vi "Instrument fgv.vi"(7 "Enum":T1(ring), 8 "error in (no error) 2":errorcluster, 10 "WriteCC1":string[](array[string])=[""], 11 "INPUT":T2) -> (0 "error":errorcluster, 2 "WriteCC1 2":string[](array[string]), 3 "output":T2)   [LabVIEW 2025]
uses:
  40ab9981-9a43-4b6a-897e-d3960d716397.vi
  <vilib>/Utility/error.llb/Trim Whitespace One-Sided.vi
  <vilib>/Instr/_visa.llb/VISA Configure Serial Port (Instr).vi
panel:
  out "trimmed string":string
  out "error out 3":errorcluster
  out "error out":errorcluster
  out "Serial Settings:Number of Bytes at Serial Port":u32
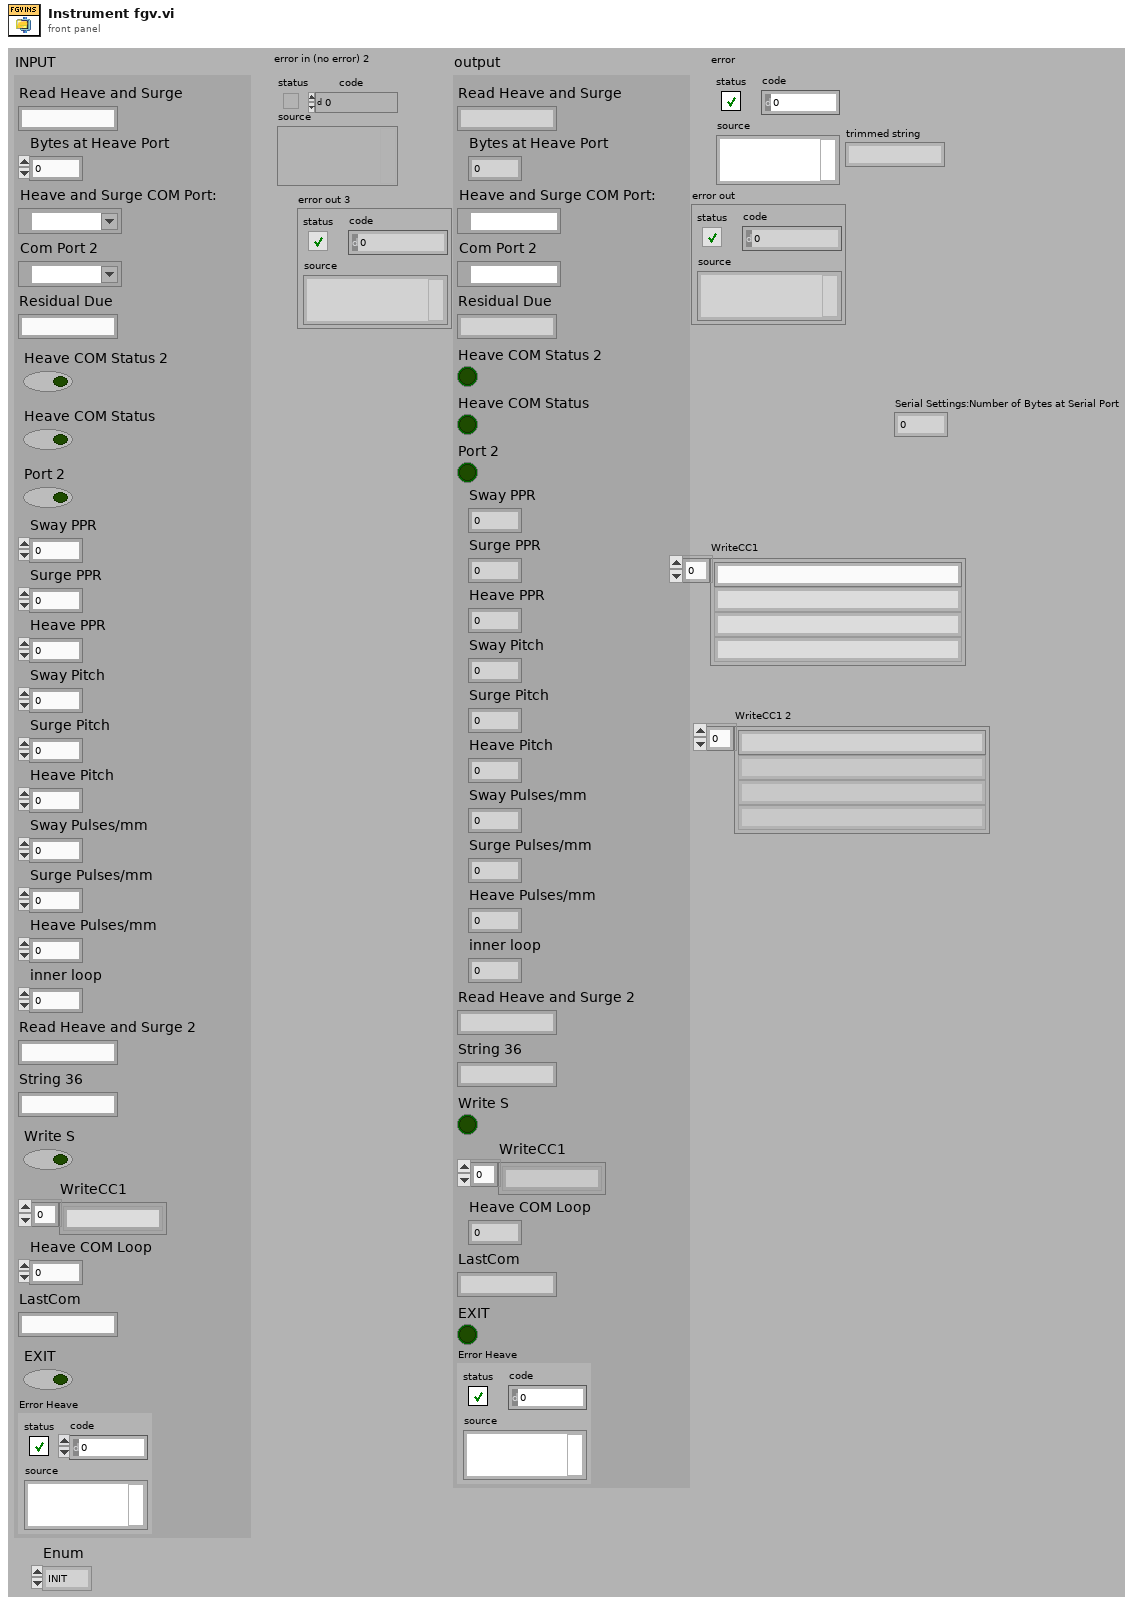
[diagram p1: front panel]
types:
  T1 = enum16{"INIT", "READ", "MANUAL WRITE", "WRITE", "CLOSE", "ERROR INIT"}
  T2 = cluster{"Read Heave and Surge":string, "Bytes at Heave Port":dbl, "Heave and Surge COM Port:":refnum<visa-resource-name>, "Com Port 2":refnum<visa-resource-name>, "Residual Due":string, "Heave COM Status 2":bool, "Heave COM Status":bool, "Port 2":bool, "Sway PPR":dbl, "Surge PPR":dbl, "Heave PPR":dbl, "Sway Pitch":dbl, "Surge Pitch":dbl, "Heave Pitch":dbl, "Sway Pulses/mm":dbl, "Surge Pulses/mm":dbl, "Heave Pulses/mm":dbl, "inner loop":dbl, "Read Heave and Surge 2":string, "String 36":string, "Write S":bool, "WriteCC1":string[], "Heave COM Loop":i32, "LastCom":string, "EXIT":bool, "Error Heave":errorcluster}
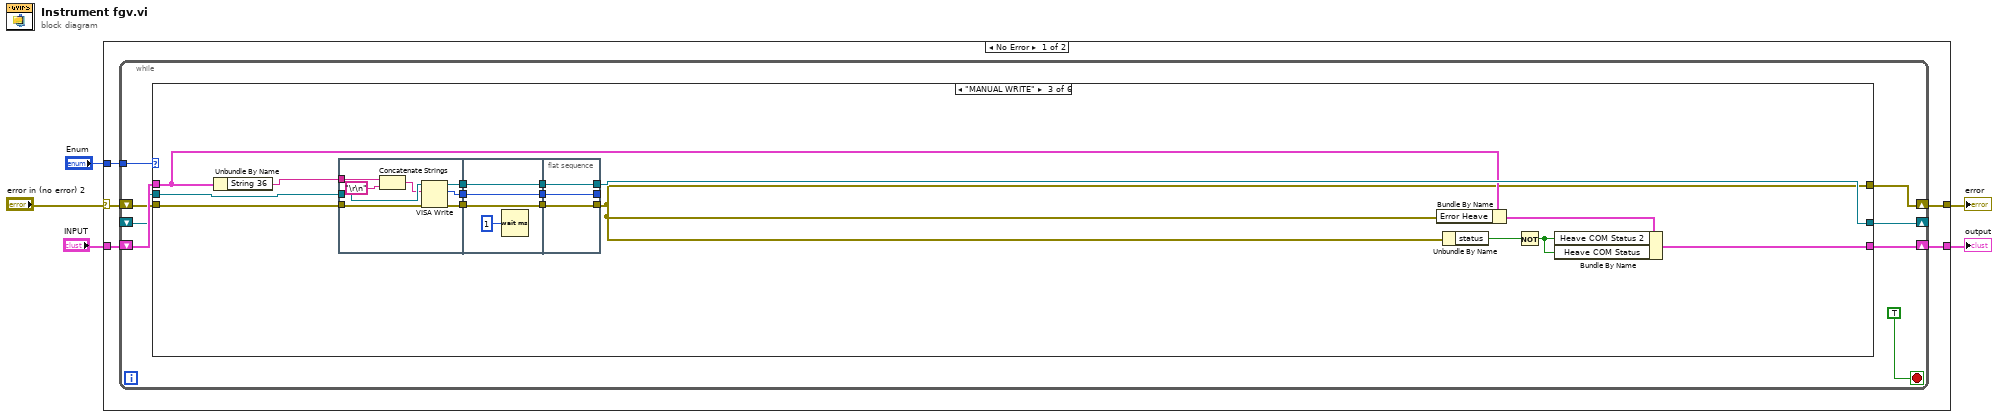
[diagram p0: block diagram]
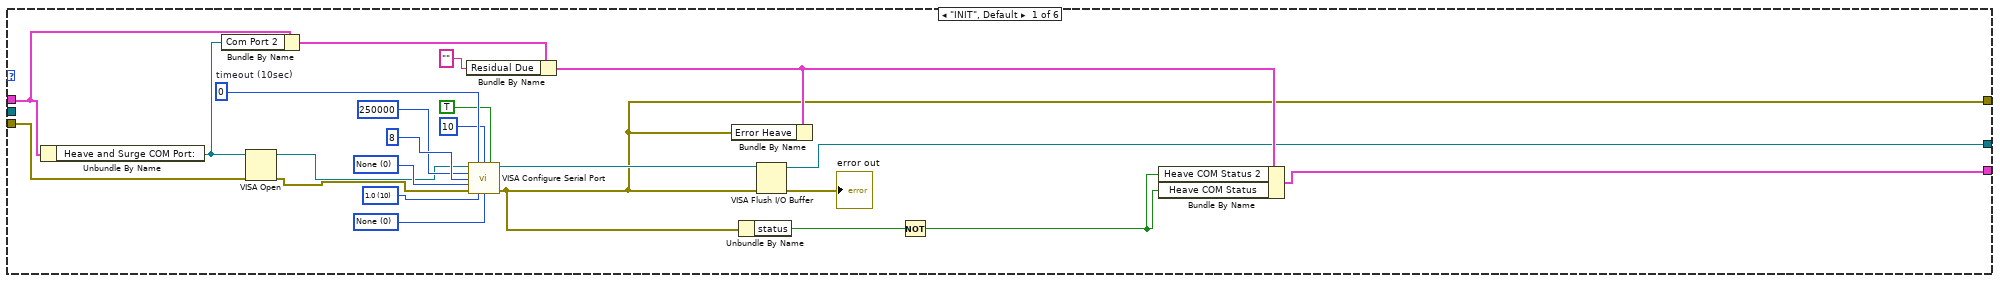
[diagram p2: hidden frame]
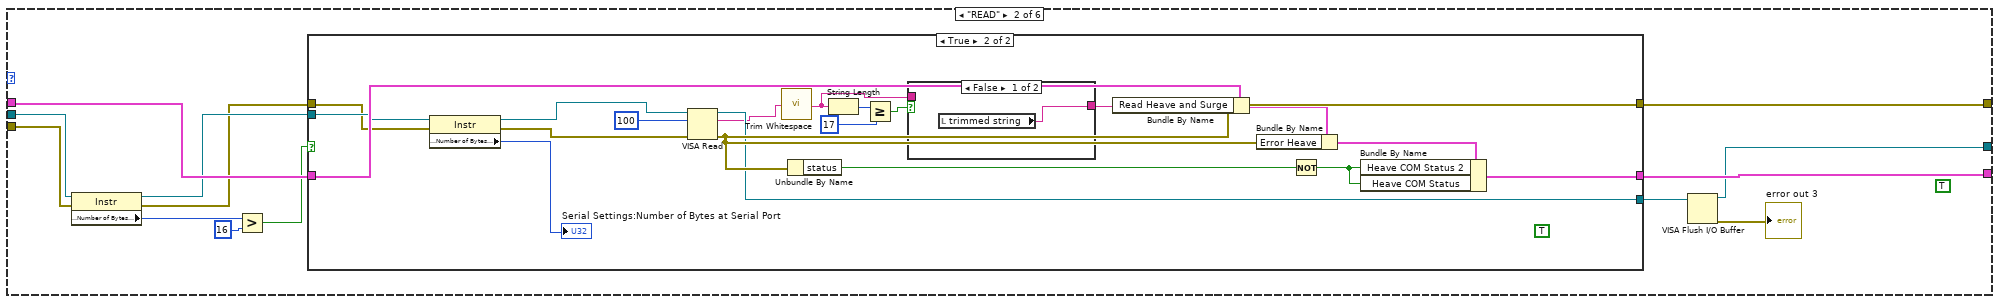
[diagram p3: hidden frame]
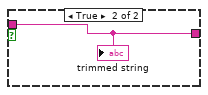
[diagram p5: hidden frame]
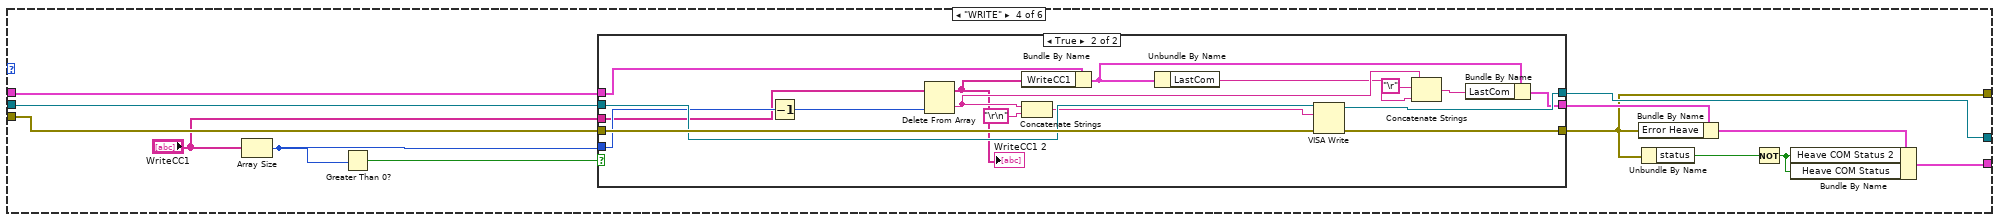
[diagram p6: hidden frame]
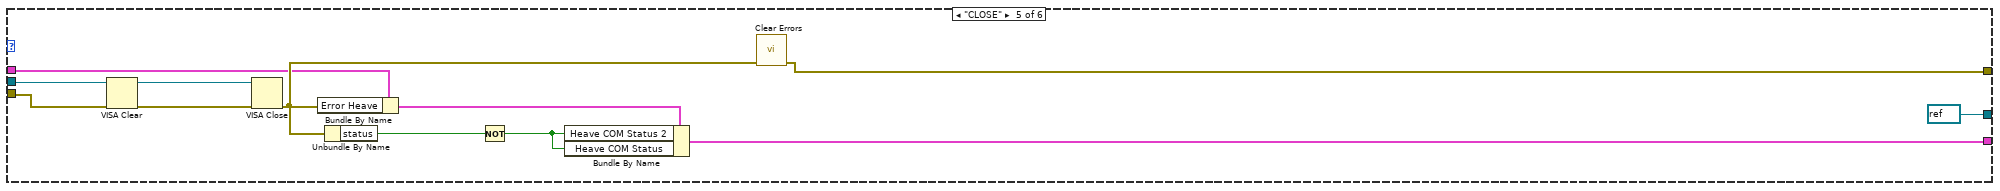
[diagram p8: hidden frame]
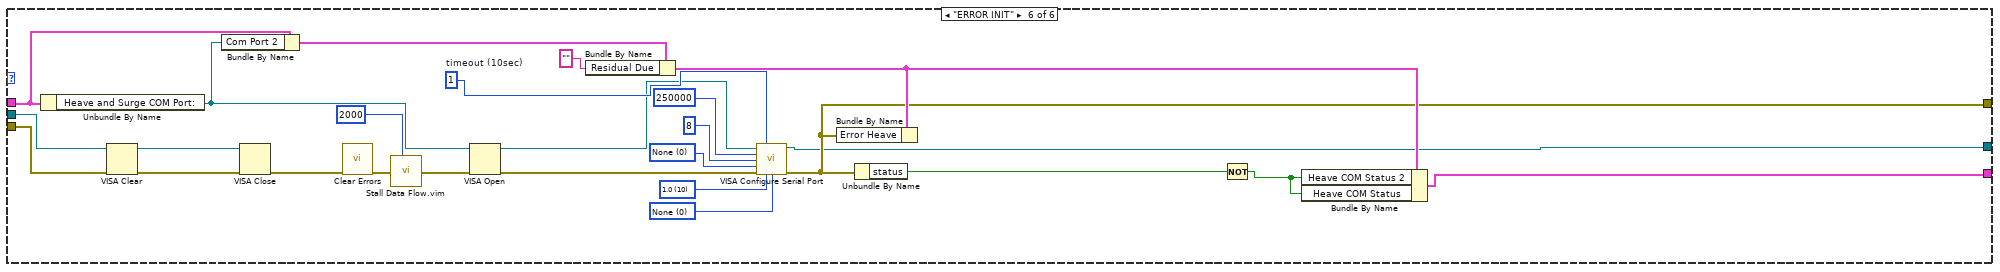
[diagram p9: hidden frame]
diagram:
  n1 = case shown="No Error" "error in (no error) 2" {
    selector: "error in (no error) 2" -> [w9 w182]
    tunnel: [w10 w182] -> w2
    tunnel: "Enum" -> [w8 _]
    tunnel: "INPUT" -> [w7 w183]
    tunnel: [w6 w183] -> w5
    frame No Error {
      n2 = while {
        tunnel: w8 -> [w17]
        shift-right: [w13] -> w10
        shift-left: w9 -> [w14]
        shift-right: [w16] -> w6
        shift-left: w7 -> [w15]
        shift-right: [w12] -> _
        shift-left: _ -> [w11]
        stop <- TRUE ("stop 3") stop-if-true
        n3 = case shown="\"MANUAL WRITE\"" w17 {
          tunnel: [w30 w53 w81 w115 w145 w158] -> w16
          tunnel: w15 -> [w26 w54 w83 w118 w146 w162]
          tunnel: w14 -> [w27 w45 w87 w120 w153 w178]
          tunnel: [w22 w52 w82 w114 w151 w160] -> w13
          tunnel: [w23 w50 w88 w119 refnum<visa-resource-name> refnum ("duplicate VISA resource name") w159] -> w12
          tunnel: w11 -> [_ w46 w89 w121 w152 w177]
          frame "INIT", Default {
            w40 = u16 0 items=["None", "XON/XOFF", "RTS/CTS", "XON/XOFF & RTS/CTS", "DTR/DSR", "XON/XOFF & DTR/DSR"] ("flow control (0:none)  2")
            w38 = u16 10 items=["1.0"=10, "1.5"=15, "2.0"=20] ("stop bits 2")
            w37 = u16 0 items=["None", "Odd", "Even", "Mark", "Space"] ("parity 2")
            w35 = u32 0  # timeout (10sec)
            n4 = Unbundle By Name(w26) -> ("Heave and Surge COM Port:"=w24:refnum<visa-resource-name>)
            n5 = Bundle By Name(cluster=w26, "Com Port 2"=w24) -> (w25:T2)
            n6 = VISA Open(error in (no error)=w27, VISA resource name=w24) -> (VISA resource name=w33:refnum<visa-resource-name>, error out=w34:errorcluster)  [unwired: 3 in]
            n7 = Bundle By Name(cluster=w25, "Residual Due"="") -> (w31:T2)
            n8 = call-poly "VISA Configure Serial Port"("VISA resource name"=w33, "timeout (10sec)"=w35, "termination char\n(0xA = '\\n' = LF)"=u8 10 ("termination char\n(0xA = '\\n' = LF)"), "Enable Termination\nChar (T)"=TRUE ("Enable Termination\nChar (T)"), "baud rate (9600)"=u32 250000 ("baud rate  2"), "data bits (8)"=u16 8 ("data bits  2"), "parity (0:none)"=w37, "error in (no error)"=w34, "stop bits (10: 1 bit)"=w38, "flow control (0:none)"=w40) -> ("VISA resource name out"=w32:refnum<visa-resource-name>, "error out"=w22:errorcluster)  [unwired: 4 in]
            n9 = Bundle By Name(cluster=w31, "Error Heave"=w22) -> ()  [unwired: 1 out]
            n10 = Unbundle By Name(w22) -> ("status"=w29:bool)
            n11 = VISA Flush I/O Buffer(VISA resource name=w32, error in (no error)=w22) -> (VISA resource name out=w23:refnum<visa-resource-name>, error out=→"error out":errorcluster)  [unwired: 1 in]
            n12 = Not(x=w29) -> (.not. x?=w28:bool)
            n13 = Bundle By Name(cluster=w31, "Heave COM Status 2"=w28, "Heave COM Status"=w28) -> (w30:T2)
          }
          frame "READ" {
            (unwired) TRUE
            n14 = property class="Instr"(reference=w46, error in=w45) -> (reference out=w44:refnum<visa-resource-name>, error out=w43:errorcluster, "Serial Settings:Number of Bytes at Serial Port"=w47:u32)
            n15 = Greater?(x=w47, y=u32 16) -> (0:w42:bool)
            n16 = case shown="True" w42 {
              tunnel: w54 -> [w55 w77]
              tunnel: [w55 w76] -> w53
              tunnel: [w57 w75] -> w52
              tunnel: [w56 w74] -> w51
              tunnel: w44 -> [w56 w73]
              tunnel: w43 -> [w57 w72]
              frame False {
              }
              frame True {
                (unwired) TRUE
                n17 = property class="Instr"(reference=w73, error in=w72) -> (reference out=w66:refnum<visa-resource-name>, error out=w65:errorcluster, "Serial Settings:Number of Bytes at Serial Port"=→"Serial Settings:Number of Bytes at Serial Port":u32)
                n18 = VISA Read(VISA resource name=w66, byte count=u32 100, error in (no error)=w65) -> (VISA resource name out=w74:refnum<visa-resource-name>, read buffer=w63:string, error out=w75:errorcluster)  [unwired: 1 out]
                n19 = call <vilib>:"Trim Whitespace.vi"("string"=w63) -> ("trimmed string"=w58:string)  [unwired: 1 in]
                n20 = Unbundle By Name(w75) -> ("status"=w69:bool)
                n21 = String Length(string=w58) -> (length=w62:i32)
                n22 = Greater Or Equal?(x=w62, y=17) -> (x >= y?=w60:bool)
                n23 = case shown="False" w60 {
                  tunnel: [w78 w79] -> w59
                  tunnel: w58 -> [_ w79]
                  frame False {
                    n24 = local read "trimmed string"() -> (w78:string)
                  }
                  frame True {
                    "trimmed string" <- w79
                  }
                }
                n25 = Bundle By Name(cluster=w77, "Read Heave and Surge"=w59) -> (w71:T2)
                n26 = Bundle By Name(cluster=w71, "Error Heave"=w75) -> (w70:T2)
                n27 = Not(x=w69) -> (.not. x?=w68:bool)
                n28 = Bundle By Name(cluster=w70, "Heave COM Status 2"=w68, "Heave COM Status"=w68) -> (w76:T2)
              }
            }
            n29 = VISA Flush I/O Buffer(VISA resource name=w51) -> (VISA resource name out=w50:refnum<visa-resource-name>, error out=→"error out 3":errorcluster)  [unwired: 2 in]
          }
          frame "MANUAL WRITE" {
            n30 = Unbundle By Name(w83) -> ("String 36"=w86:string)
            n31 = flat-sequence {
              tunnel: w89 -> [w100]
              tunnel: w87 -> [w99]
              tunnel: w86 -> [w98]
              tunnel: [w103] -> w95
              tunnel: [w102] -> w94
              tunnel: [w101] -> w93
              tunnel: w95 -> [w107]
              tunnel: w94 -> [w106]
              tunnel: w93 -> [w105]
              tunnel: [w107] -> w92
              tunnel: [w106] -> w91
              tunnel: [w105] -> w90
              tunnel: [w108] -> _
              tunnel: [w109] -> w82
              tunnel: [w110] -> w88
              tunnel: w92 -> [w110]
              tunnel: w91 -> [w109]
              tunnel: w90 -> [w108]
              frame #0 {
                n32 = Concatenate Strings(w98, "\r\n") -> (w97:string)
                n33 = VISA Write(VISA resource name=w100, write buffer=w97, error in (no error)=w99) -> (VISA resource name out=w103:refnum<visa-resource-name>, return count=w101:u32, error out=w102:errorcluster)
              }
              frame #1 {
                n34 = Wait (ms)(milliseconds to wait=u32 1) -> ()  [unwired: 1 out]
              }
              frame #2 {
              }
            }
            n35 = Bundle By Name(cluster=w83, "Error Heave"=w82) -> (w85:T2)
            n36 = Unbundle By Name(w82) -> ("status"=w84:bool)
            n37 = Not(x=w84) -> (.not. x?=w80:bool)
            n38 = Bundle By Name(cluster=w85, "Heave COM Status 2"=w80, "Heave COM Status"=w80) -> (w81:T2)
          }
          frame "WRITE" {
            n39 = Array Size(array="WriteCC1") -> (size(s)=w123:i32)
            n40 = Greater Than 0?(x=w123) -> (x > 0?=w122:bool)
            n41 = case shown="True" w122 {
              tunnel: [w126 w136] -> w114
              tunnel: w120 -> [w126 w142]
              tunnel: [w125 w140] -> w119
              tunnel: w121 -> [w125 w141]
              tunnel: "WriteCC1" -> [_ w137]
              tunnel: w123 -> [_ w139]
              tunnel: w118 -> [w124 w133]
              tunnel: [w124 w130] -> w117
              frame False {
              }
              frame True {
                n42 = Decrement(x=w139) -> (x-1=w138:i32)
                n43 = Delete From Array(array=w137, index=w138) -> (deleted portion=w135:string, array with subset deleted=w129:string[])  [unwired: 1 in]
                "WriteCC1 2" <- w129
                n44 = Bundle By Name(cluster=w133, "WriteCC1"=w129) -> (w132:T2)
                n45 = Concatenate Strings(w135, "\r\n") -> (w128:string)
                n46 = Unbundle By Name(w132) -> ("LastCom"=w131:string)
                n47 = VISA Write(VISA resource name=w141, write buffer=w128, error in (no error)=w142) -> (VISA resource name out=w140:refnum<visa-resource-name>, error out=w136:errorcluster)  [unwired: 1 out]
                n48 = Concatenate Strings(w135, "\r", w131) -> (w134:string)
                n49 = Bundle By Name(cluster=w132, "LastCom"=w134) -> (w130:T2)
              }
            }
            n50 = Bundle By Name(cluster=w117, "Error Heave"=w114) -> (w116:T2)
            n51 = Unbundle By Name(w114) -> ("status"=w113:bool)
            n52 = Not(x=w113) -> (.not. x?=w112:bool)
            n53 = Bundle By Name(cluster=w116, "Heave COM Status 2"=w112, "Heave COM Status"=w112) -> (w115:T2)
          }
          frame "CLOSE" {
            n54 = VISA Clear(VISA resource name=w152, error in (no error)=w153) -> (VISA resource name out=w155:refnum<visa-resource-name>, error out=w154:errorcluster)
            n55 = VISA Close(VISA resource name=w155, error in (no error)=w154) -> (error out=w147:errorcluster)
            n56 = Bundle By Name(cluster=w146, "Error Heave"=w147) -> (w150:T2)
            n57 = Unbundle By Name(w147) -> ("status"=w149:bool)
            n58 = Not(x=w149) -> (.not. x?=w148:bool)
            n59 = Bundle By Name(cluster=w150, "Heave COM Status 2"=w148, "Heave COM Status"=w148) -> (w145:T2)
            n60 = call <vilib>:"Clear Errors.vi"("error in (no error)"=w147) -> ("error out"=w151:errorcluster)  [unwired: 5 in, 1 out]
          }
          frame "ERROR INIT" {
            w175 = u16 0 items=["None", "XON/XOFF", "RTS/CTS", "XON/XOFF & RTS/CTS", "DTR/DSR", "XON/XOFF & DTR/DSR"] ("flow control (0:none)  2")
            w173 = u16 10 items=["1.0"=10, "1.5"=15, "2.0"=20] ("stop bits 2")
            w172 = u16 0 items=["None", "Odd", "Even", "Mark", "Space"] ("parity 2")
            w170 = u32 1  # timeout (10sec)
            n61 = Unbundle By Name(w162) -> ("Heave and Surge COM Port:"=w163:refnum<visa-resource-name>)
            n62 = VISA Clear(VISA resource name=w177, error in (no error)=w178) -> (VISA resource name out=w181:refnum<visa-resource-name>, error out=w180:errorcluster)
            n63 = Bundle By Name(cluster=w162, "Com Port 2"=w163) -> (w164:T2)
            n64 = VISA Close(VISA resource name=w181, error in (no error)=w180) -> (error out=w179:errorcluster)
            n65 = call <vilib>:"Clear Errors.vi"("error in (no error)"=w179) -> ("error out"=w161:errorcluster)  [unwired: 5 in, 1 out]
            n66 = call "Stall Data Flow.vim"("value in"=w161, "milliseconds to wait"=u32 2000) -> ("value out"=w157:errorcluster)  [unwired: 1 out]
            n67 = VISA Open(error in (no error)=w157, VISA resource name=w163) -> (VISA resource name=w168:refnum<visa-resource-name>, error out=w169:errorcluster)  [unwired: 3 in]
            n68 = Bundle By Name(cluster=w164, "Residual Due"="") -> (w167:T2)
            n69 = call-poly "VISA Configure Serial Port"("VISA resource name"=w168, "timeout (10sec)"=w170, "baud rate (9600)"=u32 250000 ("baud rate  2"), "data bits (8)"=u16 8 ("data bits  2"), "parity (0:none)"=w172, "error in (no error)"=w169, "stop bits (10: 1 bit)"=w173, "flow control (0:none)"=w175) -> ("VISA resource name out"=w159:refnum<visa-resource-name>, "error out"=w160:errorcluster)  [unwired: 6 in]
            n70 = Bundle By Name(cluster=w167, "Error Heave"=w160) -> ()  [unwired: 1 out]
            n71 = Unbundle By Name(w160) -> ("status"=w166:bool)
            n72 = Not(x=w166) -> (.not. x?=w165:bool)
            n73 = Bundle By Name(cluster=w167, "Heave COM Status 2"=w165, "Heave COM Status"=w165) -> (w158:T2)
          }
        }
      }
    }
    frame Error {
    }
  }
  "output" <- w5
  "error" <- w2
